vi "Initialize SLSC Module.vi"(8 "error in (no error)":errorcluster, 9 "SLSC Custom Device Information":T1 {"Custom Device Information"."Dependencies"."Type" items=["Absolute", "ToBase", "ToCommonDocDir", "ToApplicationDataDir"]; "Custom Device Information"."Driver VIs"."Type" items=["Absolute", "ToBase", "ToCommonDocDir", "ToApplicationDataDir"]; "Custom Device Information"."Execution Mode" items=["Asynchronous", "InlineHWInterface", "InlineModelInterface", "InlineTimingandSync", "AsynchronousTimingandSync"]}, 10 "Name":string, 11 "SLSC Module":u64) -> (0 "error out":errorcluster, 3 "SLSC Module out":u64)   [LabVIEW 2020, in "VeriStand SLSC Scripting.lvlib"]
uses:
  VeriStand SLSC Scripting.lvlib
  Controls/SLSC Custom Device Information.ctl
  Controls/Custom Device Information.ctl
  Controls/Dependent File Information.ctl
  <vilib>/NI VeriStand/Custom Device API/Custom Device Supported Target.ctl
  NationalInstruments.VeriStand.SystemDefinitionAPI
  NationalInstruments.VeriStand.SystemStorage
  <vilib>/NI VeriStand/Custom Device API/Custom Device API.lvlib
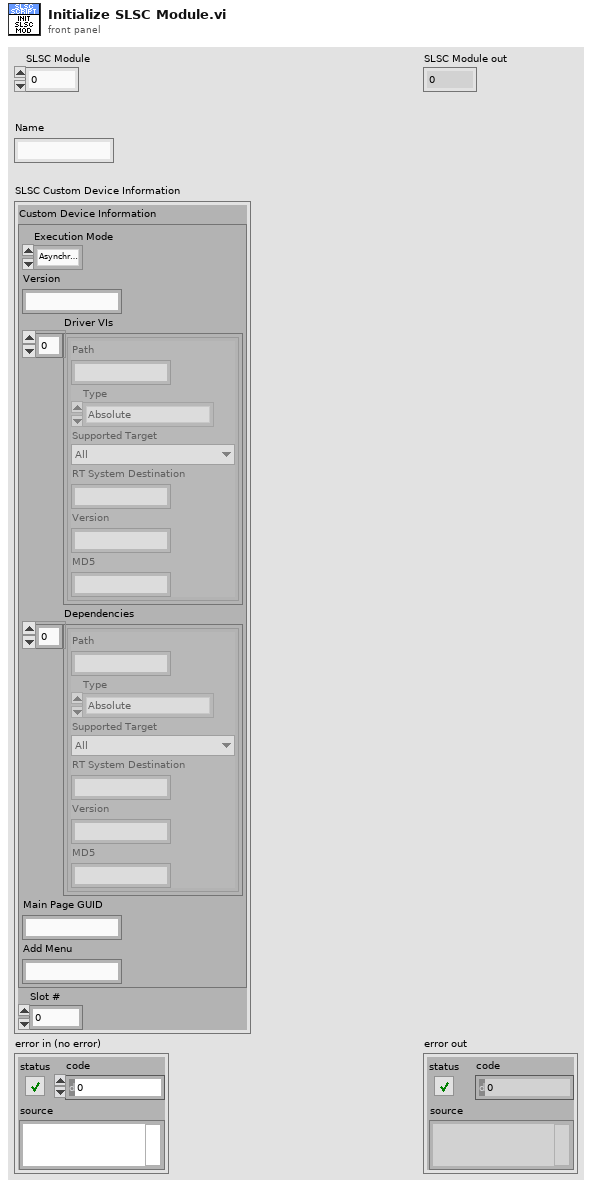
[diagram p1: front panel]
types:
  T1 = typedef "VeriStand SLSC Scripting.lvlib/SLSC Custom Device Information.ctl" = cluster{"Custom Device Information":T2, "Slot #":i32}
  T2 = typedef "VeriStand SLSC Scripting.lvlib/Custom Device Information.ctl" = cluster{"Execution Mode":i32, "Version":string, "Driver VIs":T3[], "Dependencies":T3[], "Main Page GUID":string, "Add Menu":string}
  T3 = typedef "VeriStand SLSC Scripting.lvlib/Dependent File Information.ctl" = cluster{"Path":string, "Type":i32, "Supported Target":T4, "RT System Destination":string, "Version":string, "MD5":string}
  T4 = typedef "Custom Device API.lvlib/Custom Device Supported Target.ctl" = enum16{"All", "PharLap", "VxWorks", "Windows", "Linux_32_ARM", "Linux_x64", "PharLap & Windows", "PharLap & VxWorks", "VxWorks & Windows"}
  T5 = cluster{"Property Name Format String":string, "Offset":i32, "Reverse Order":bool}
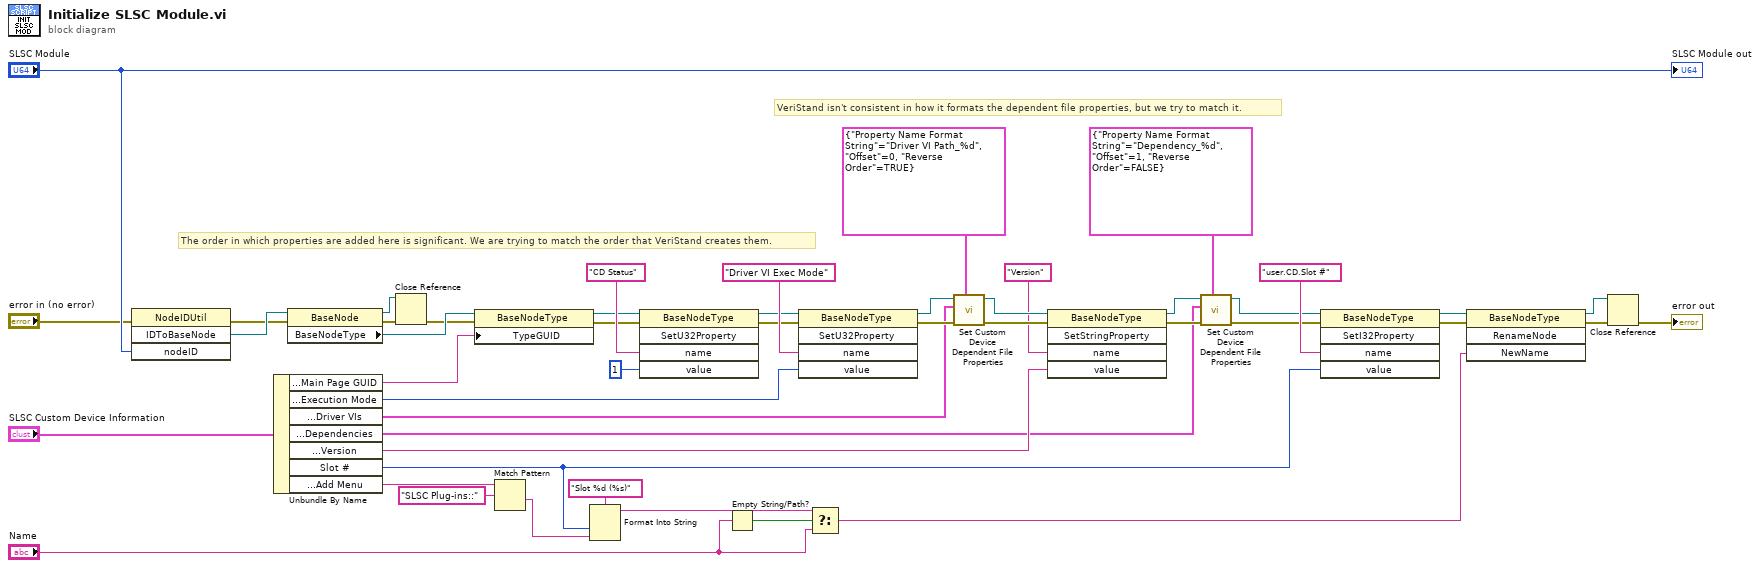
[diagram p0: block diagram]
diagram:
  # "The order in which properties are added here is significant. We are trying to match the order that VeriStand creates them."
  # "VeriStand isn't consistent in how it formats the dependent file properties, but we try to match it."
  n1 = invoke class="NodeIDUtil" method="IDToBaseNode"(error in="error in (no error)", "nodeID"="SLSC Module") -> (error out=w24:errorcluster, "IDToBaseNode"=w25:refnum<k24>)  [unwired: 2 in, 2 out]
  n2 = Unbundle By Name("SLSC Custom Device Information") -> ("Custom Device Information.Main Page GUID"=w45:string, "Custom Device Information.Execution Mode"=w37:i32, "Custom Device Information.Driver VIs"=w34:T3[], "Custom Device Information.Dependencies"=w4:T3[], "Custom Device Information.Version"=w32:string, "Slot #"=w18:i32, "Custom Device Information.Add Menu"=w13:string)
  n3 = property class="BaseNode"(reference=w25, error in=w24) -> (reference out=w29:refnum<k24>, error out=w47:errorcluster, "BaseNodeType"=w27:refnum<k24>)
  n4 = Close Reference(reference=w29, error in (no error)=w47) -> (error out=w26:errorcluster)
  n5 = property class="BaseNodeType"(reference=w27, error in=w26, "TypeGUID"=w45) -> (reference out=w38:refnum<k24>, error out=w39:errorcluster)
  n6 = Match Pattern(string=w13, regular expression="SLSC Plug-ins::") -> (after substring=w11:string)  [unwired: 1 in, 3 out]
  n7 = Format Into String(format string="Slot %d (%s)", w18, w11) -> (resulting string=w15:string)  [unwired: 2 in, 1 out]
  n8 = invoke class="BaseNodeType" method="SetU32Property"(reference=w38, error in=w39, "name"="CD Status", "value"=u32 1) -> (reference out=w40:refnum<k24>, error out=w41:errorcluster)  [unwired: 1 in, 3 out]
  n9 = Empty String/Path?(string/path="Name") -> (empty?=w17:bool)
  n10 = invoke class="BaseNodeType" method="SetU32Property"(reference=w40, error in=w41, "name"="Driver VI Exec Mode", "value"=w37) -> (reference out=w35:refnum<k24>, error out=w36:errorcluster)  [unwired: 1 in, 3 out]
  n11 = Select(t=w15, s=w17, f="Name") -> (s? t:f=w14:string)
  n12 = call "Set Custom Device Dependent File Properties.vi"("Format Settings"=T5 {"Property Name Format String"="Driver VI Path_%d", "Offset"=0, "Reverse Order"=TRUE}, "error in (no error)"=w36, "Dependent Files"=w34, "BaseNodeType"=w35) -> ("error out"=w8:errorcluster, "BaseNodeType out"=w7:refnum<k24>)  [unwired: 6 in]
  n13 = invoke class="BaseNodeType" method="SetStringProperty"(reference=w7, error in=w8, "name"="Version", "value"=w32) -> (reference out=w6:refnum<k24>, error out=w5:errorcluster)  [unwired: 1 in, 3 out]
  n14 = call "Set Custom Device Dependent File Properties.vi"("Format Settings"=T5 {"Property Name Format String"="Dependency_%d", "Offset"=1, "Reverse Order"=FALSE}, "error in (no error)"=w5, "Dependent Files"=w4, "BaseNodeType"=w6) -> ("error out"=w2:errorcluster, "BaseNodeType out"=w1:refnum<k24>)  [unwired: 6 in]
  n15 = invoke class="BaseNodeType" method="SetI32Property"(reference=w1, error in=w2, "name"="user.CD.Slot #", "value"=w18) -> (reference out=w22:refnum<k24>, error out=w23:errorcluster)  [unwired: 1 in, 3 out]
  n16 = invoke class="BaseNodeType" method="RenameNode"(reference=w22, error in=w23, "NewName"=w14) -> (reference out=w20:refnum<k24>, error out=w21:errorcluster)  [unwired: 1 in, 2 out]
  n17 = Close Reference(reference=w20, error in (no error)=w21) -> (error out=→"error out":errorcluster)
  "SLSC Module out" <- "SLSC Module"
